vi "浮点转DCBA整形.vi"(11 "浮点数":sgl[](array[numeric])) -> (3 "DCBA整形输出":u16[](array[numeric]) format="%04xH")   [LabVIEW 2016]
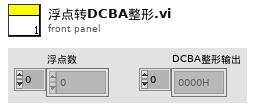
[diagram p1: front panel]
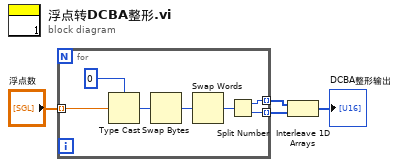
[diagram p0: block diagram]
diagram:
  n1 = for {
    tunnel: "浮点数" -> [w7] mode=indexing
    tunnel: [w6] -> w2 mode=indexing
    tunnel: [w5] -> w3 mode=indexing
    n2 = Type Cast(type=0, x=w7) -> (*(type *) &x=w9:i32)
    n3 = Swap Bytes(anything=w9) -> (byte swapped=w8:i32)
    n4 = Swap Words(1:w8) -> (0:w11:i32)
    n5 = Split Number(x=w11) -> (hi(x)=w6:u16, lo(x)=w5:u16)
  }
  n6 = Interleave 1D Arrays(w2, w3) -> (→"DCBA整形输出":u16[])
